vi "getSerializedData.vi"(0 "reference":refnum<class "PointNode.lvclass">, 5 "error in (no error)":errorcluster) -> (14 "reference out":refnum<class "PointNode.lvclass">, 15 "parent":refnum<class "AbstractNode.lvclass">, 16 "children":refnum<class "AbstractNode.lvclass">[](array[class]), 17 "xmlOut":string, 19 "error out":errorcluster)   [LabVIEW 2014, in "PointNode.lvclass"]
doc: "getSerializedData"
uses:
  <resource>/Framework/Providers/Open_GDS/UML/PointNode_class/PointNode.lvclass
  <resource>/Framework/Providers/Open_GDS/UML/AbstractNode_class/AbstractNode.lvclass
  <resource>/Framework/Providers/Open_GDS/UML/AbstractNode_class/ObjectReference.ctl
  <resource>/Framework/Providers/Open_GDS/UML/General/Point/Point Point2D.ctl
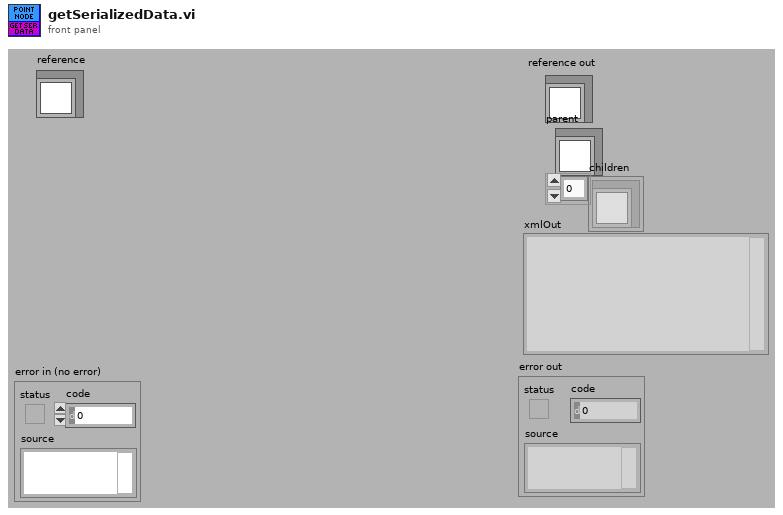
[diagram p1: front panel]
types:
  T1 = typedef "AbstractNode.lvclass/ObjectReference.ctl" = refnum<k1>
  T2 = typedef "Point Point2D.ctl" = cluster{"x":dbl, "y":dbl}
  T3 = cluster{"Base class":cluster{"parent":T1, "children":T1[]}, "point":T2}
  T4 = typedef "PointNode.lvclass/ObjectAttributes.ctl" = cluster{"Base class":T5, "point":T2}
  T5 = typedef "AbstractNode.lvclass/ObjectAttributes.ctl" = cluster{"parent":refnum<class "AbstractNode.lvclass">, "children":refnum<class "AbstractNode.lvclass">[], "Hidden":bool}
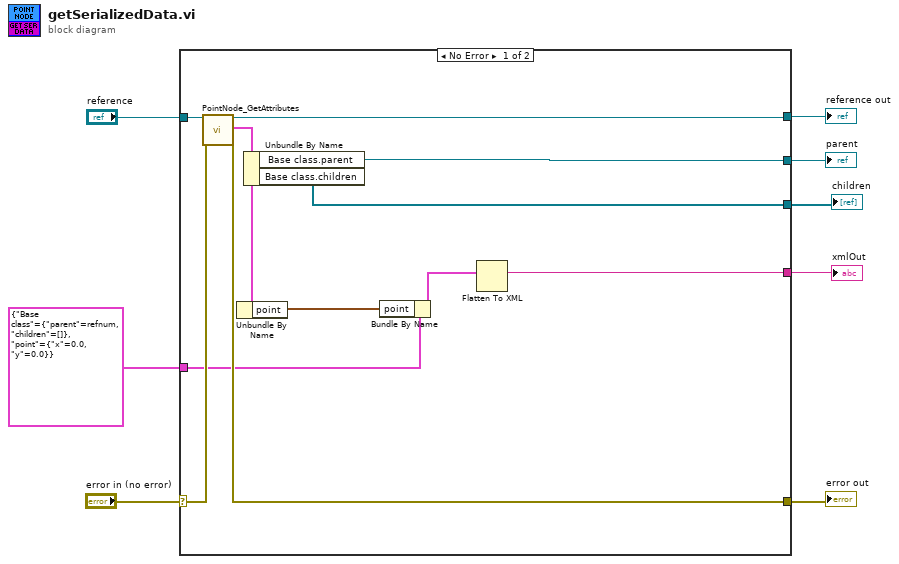
[diagram p0: block diagram]
diagram:
  n1 = case shown="No Error" "error in (no error)" {
    selector: "error in (no error)" -> [w19 w20]
    tunnel: "reference" -> [w18 w21]
    tunnel: [w16 w20] -> w6
    tunnel: [w17 w21] -> w5
    tunnel: [w15 _] -> w4
    tunnel: [w14 _] -> w3
    tunnel: [w13 _] -> w2
    tunnel: T3 {"Base class"={"parent"=refnum, "children"=[]}, "point"={"x"=0.0, "y"=0.0}} ("Attributes") -> [w11 _]
    frame No Error {
      n2 = call <resource>:"PointNode_GetAttributes.vi"("reference in"=w18, "error in (no error)"=w19) -> ("reference out"=w17:refnum<class "PointNode.lvclass">, "Attributes"=w12:T4, "error out"=w16:errorcluster)  [unwired: 15 out]
      n3 = Unbundle By Name(w12) -> ("point"=w10:T2)
      n4 = Unbundle By Name(w12) -> ("Base class.parent"=w15:refnum<class "AbstractNode.lvclass">, "Base class.children"=w14:refnum<class "AbstractNode.lvclass">[])
      n5 = Bundle By Name(cluster=w11, "point"=w10) -> (w9:T3)
      n6 = Flatten To XML(anything=w9) -> (xml string=w13:string)
    }
    frame Error {
    }
  }
  "reference out" <- w5
  "error out" <- w6
  "parent" <- w4
  "children" <- w3
  "xmlOut" <- w2
